vi "FRCts20_Backend_INI_Close.vi"(8 "error in (no error)":errorcluster, 11 "INI Controller in":refnum<class "FRCts20_Backend_INI Controller.lvclass">) -> (0 "error out":errorcluster, 2 "file path":path, 3 "INI Controller out":refnum<class "FRCts20_Backend_INI Controller.lvclass">)   [LabVIEW 2014, in "FRCts20_Backend_Engine.lvlib" / "FRCts20_Backend_INI Controller.lvclass"]
uses:
  FRCts20_Backend_INI Controller.lvclass
  FRCts20_Backend_INI Controller.lvclass/FRCts20_Backend_INI Controller.ctl
  <vilib>/Utility/config.llb/NI_LVConfig.lvlib
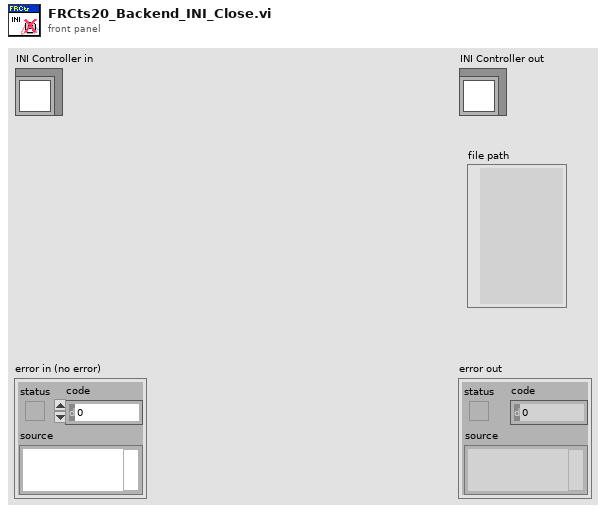
[diagram p1: front panel]
types:
  T1 = typedef "NI_LVConfig.lvlib/Config Data RefNum.ctl" = refnum<k1>
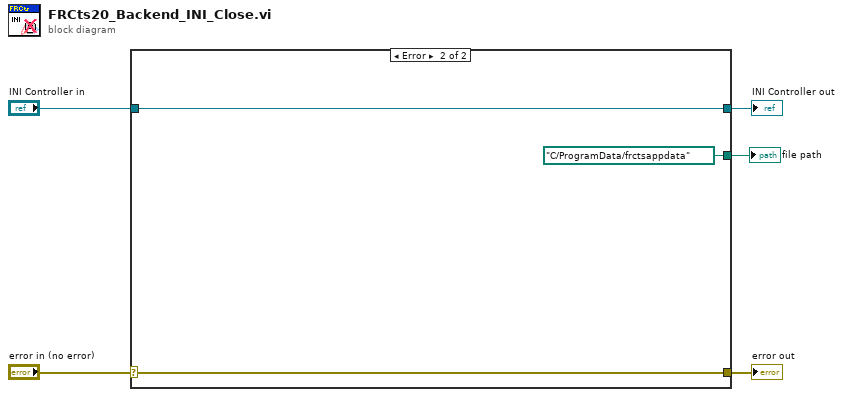
[diagram p0: block diagram]
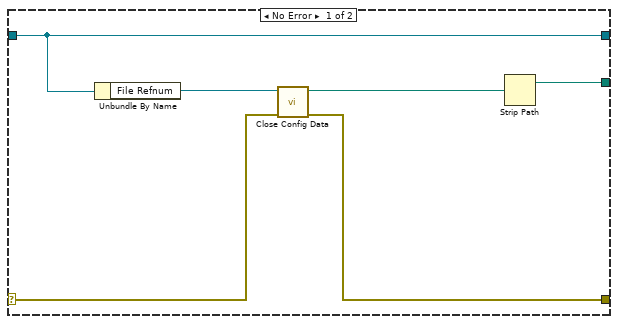
[diagram p2: hidden frame]
diagram:
  n1 = case shown="Error" "error in (no error)" {
    selector: "error in (no error)" -> [w9 w14]
    tunnel: [w10 w14] -> w4
    tunnel: [w6 w13] -> w2
    tunnel: "INI Controller in" -> [w6 w13]
    tunnel: [w7 path "C:/ProgramData/frctsappdata" ("stripped path")] -> w1
    frame No Error {
      n2 = Unbundle By Name(w6) -> ("File Refnum"=w11:T1)
      n3 = call <vilib>:"Close Config Data.vi"("error in (no error)"=w9, "refnum"=w11) -> ("error out"=w10:errorcluster, "file path"=w8:path)  [unwired: 8 in]
      n4 = Strip Path(path=w8) -> (stripped path=w7:path)  [unwired: 1 out]
    }
    frame Error {
    }
  }
  "error out" <- w4
  "INI Controller out" <- w2
  "file path" <- w1
